vi "PixelAtDistanceR.vi"(1 "R (innner)":dbl, 2 "R (including)":dbl=22.0) -> (0 "XY-Graph":cdb[](graph))   [LabVIEW 2011]
panel:
  out "Geschätzte Elemete":dbl
  out "Größe(n)":i32
  # "Pixelfolge im Abstand R, Pixelraster =1 Einheit\nsollte Mindestens 1 element=00 liefern bei R-inner =0"
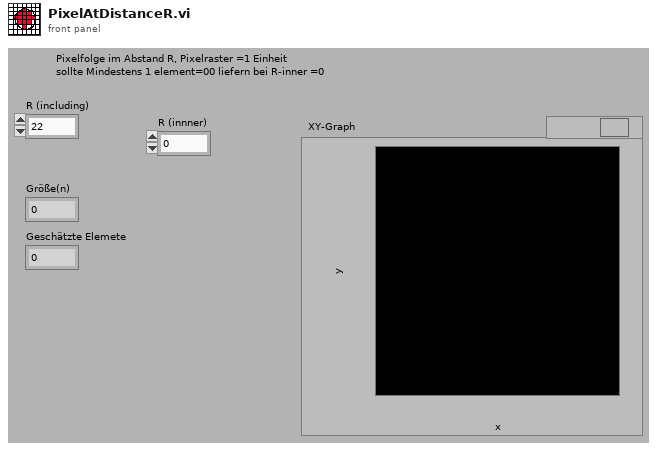
[diagram p1: front panel]
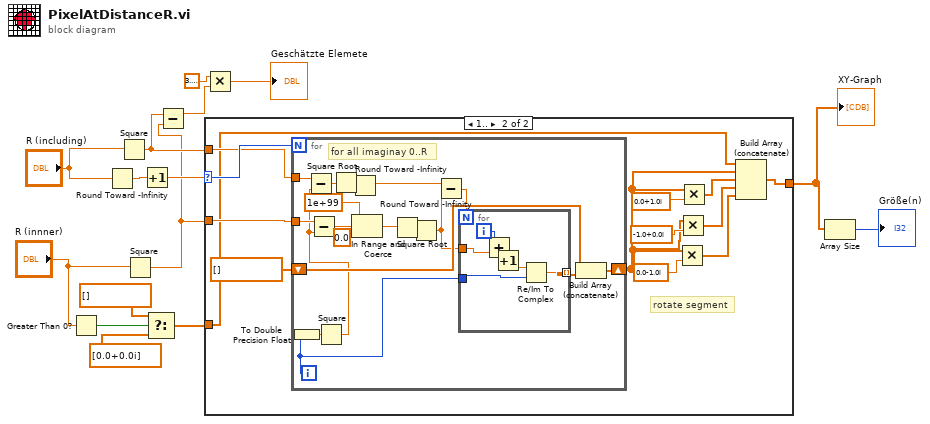
[diagram p0: block diagram]
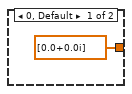
[diagram p2: hidden frame]
diagram:
  n1 = Greater Than 0?(x="R (innner)") -> (x > 0?=w4:bool)
  n2 = Round Toward -Infinity(1:"R (including)") -> (0:w14:dbl)
  n3 = Square(x="R (including)") -> (x^2=w10:dbl)
  n4 = Square(x="R (innner)") -> (x^2=w6:dbl)
  n5 = Increment(x=w14) -> (x+1=w13:dbl)
  n6 = Select(t=cdb[] [], s=w4, f=cdb[] [0.0+0.0i] ("Array")) -> (s? t:f=w1:cdb[])
  n7 = Subtract(x=w10, y=w6) -> (x-y=w7:dbl)
  n8 = Multiply(x=3.141592653589793, y=w7) -> (x*y=→"Geschätzte Elemete":dbl)
  n9 = case shown="1.." w13 {
    selector: w13 -> [_ w29]
    tunnel: w10 -> [_ w28]
    tunnel: [cdb[] [0.0+0.0i] w22] -> w12
    tunnel: w6 -> [_ w18]
    tunnel: w1 -> [_ w17]
    frame 0, Default {
    }
    frame 1.. {
      # "rotate segment"
      n10 = for {
        N: w29 -> [_]
        tunnel: w28 -> [w47]
        shift-right: [w42] -> w19
        shift-left: cdb[] [] -> [w41]
        tunnel: w18 -> [w37]
        i -> [w44]
        # "for all imaginay 0..R"
        n11 = To Double Precision Float(number=w44) -> (double precision float=w40:dbl)
        n12 = Square(x=w40) -> (x^2=w36:dbl)
        n13 = Subtract(x=w47, y=w36) -> (x-y=w46:dbl)
        n14 = Subtract(x=w37, y=w36) -> (x-y=w39:dbl)
        n15 = Square Root(x=w46) -> (sqrt(x)=w45:dbl)
        n16 = Round Toward -Infinity(1:w45) -> (0:w35:dbl)
        n17 = In Range and Coerce(upper limit=1e+99, x=w39, lower limit=0.0) -> (coerced(x)=w32:dbl)  [unwired: 1 out]
        n18 = Square Root(x=w32) -> (sqrt(x)=w38:dbl)
        n19 = Round Toward -Infinity(1:w38) -> (0:w33:dbl)
        n20 = Subtract(x=w35, y=w33) -> (x-y=w34:dbl)
        n21 = for {
          N: w34 -> [_]
          tunnel: w44 -> [w52]
          tunnel: [w51] -> w43 mode=indexing
          tunnel: w33 -> [w50]
          i -> [w49]
          n22 = Add(x=w49, y=w50) -> (x+y=w48:dbl)
          n23 = Increment(x=w48) -> (x+1=w53:dbl)
          n24 = Re/Im To Complex(1:w52, 2:w53) -> (0:w51:cdb)
        }
        n25 = Build Array (concatenate)(w41, w43) -> (w42:cdb[])
      }
      n26 = Multiply(x=w19, y=cdb 0.0-1.0i) -> (x*y=w20:cdb[])
      n27 = Multiply(x=w19, y=cdb -1.0+0.0i) -> (x*y=w21:cdb[])
      n28 = Multiply(x=w19, y=cdb 0.0+1.0i) -> (x*y=w23:cdb[])
      n29 = Build Array (concatenate)(w17, w19, w23, w21, w20) -> (w22:cdb[])
    }
  }
  "XY-Graph" <- w12
  n30 = Array Size(array=w12) -> (size(s)=→"Größe(n)":i32)
